vi "PigeonSensorReadings.vi"(1 "Reset Yaw (deg)":dbl format="%#_13g", 2 "Reset Yaw":bool) -> (0 "Yaw (deg)":dbl format="%#_13g")   [LabVIEW 2019]
doc: "This VI reads the Pigeon IMU yaw and handles error detection and orientation resets."
uses:
  refnums.vi
  <vilib>/Rock Robotics/WPI/ThirdParty/Phoenix-LabVIEW/Pigeon IMU/CTRE_PigeonIMU_GetYPR.vi
  sensors.vi
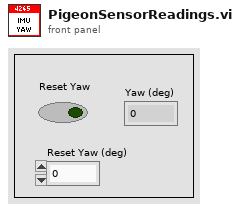
[diagram p1: front panel]
types:
  T1 = typedef "CTRE_PigeonIMU_DeviceRef.ctl" = cluster{"DeviceStatus":errorcluster, "Device Number":u8, "Type":T2, "Device ID":u32, "Handle":u64, "UsageFrame":u32, "Library Path":path}
  T2 = typedef "CTRE_PigeonIMU_ConnectionType.ctl" = u32
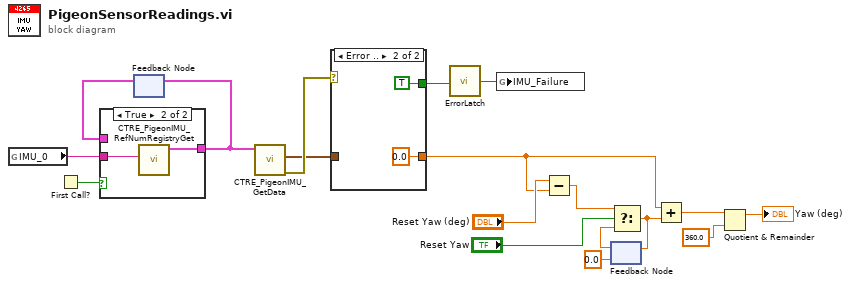
[diagram p0: block diagram]
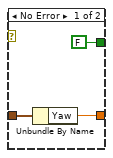
[diagram p2: hidden frame]
diagram:
  n1 = global read "refnums.vi" "IMU_0"() -> (w16:string)
  n2 = First Call?() -> (First Call?: T/F=w18:bool)
  n3 = feedback #1() -> (w17:T1)  [unwired: 1 in]
  n4 = case shown="True" w18 {
    tunnel: [w19 w21] -> w15
    tunnel: w17 -> [w19 _]
    tunnel: w16 -> [_ w20]
    frame False {
    }
    frame True {
      n5 = call <vilib>:"CTRE_PigeonIMU_RefNumRegistryGet.vi"("refnum name"=w20) -> ("PigeonIMUDevRef"=w21:T1)  [unwired: 9 in, 1 out]
    }
  }
  n6 = feedback-in #1(w15) -> ()
  n7 = call-poly <vilib>:"CTRE_PigeonIMU_GetData.vi"("PigeonIMUDevRef"=w15) -> ("error out"=w5:errorcluster, "Yaw Pitch Roll"=w2:cluster{"Yaw":dbl, "Pitch":dbl, "Roll":dbl})  [unwired: 8 in, 1 out]
  n8 = case shown="Error .." w5 {
    tunnel: [FALSE TRUE] -> w4
    tunnel: w2 -> [w23 _]
    tunnel: [w22 0.0 ("Yaw")] -> w1
    frame No Error {
      n9 = Unbundle By Name(w23) -> ("Yaw"=w22:dbl)
    }
    frame Error {
    }
  }
  n10 = call "ErrorLatch.vi"("Trigger"=w4) -> ("Latched"=w3:bool)
  n11 = global write "sensors.vi" "IMU_Failure"(w3) -> ()
  n12 = Subtract(x="Reset Yaw (deg)", y=w1) -> (x-y=w13:dbl)
  n13 = feedback #2(0.0) -> (w12:dbl)
  n14 = Select(t=w13, s="Reset Yaw", f=w12) -> (s? t:f=w10:dbl)
  n15 = feedback-in #2(w10) -> ()
  n16 = Add(x=w1, y=w10) -> (x+y=w7:dbl)
  n17 = Quotient & Remainder(x=w7, y=360.0) -> (x-y*floor(x/y)=→"Yaw (deg)":dbl)  [unwired: 1 out]
